vi "PIM Driver.vi"(5 "PIM Driver Name/Configuration":string, 6 "Driver Ref (null)":T1, 7 "PIM Command":T11, 8 "error in (no error)":errorcluster, 11 "Stimulus":T3={"Carrier Frequencies"={"C1 Freq, MHz"=0.0, "C2 Freq, MHz"=0.0}, "Carrier Powers"={"C1 Power,dBm"=0.0, "C2 Power, dBm"=0.0}, "Measurement Parameters"={"IM Order"=0, "Averaging"=1, "Direction"=0, "Enable ALC?"=FALSE, "Enable SingleIM?"=FALSE, "Display Units"=enum."dBm", "VA Hold?"=FALSE, "DUT PORT"=enum."Port 1"}, "Measurement Setup"={"Meas Type"=enum."Time", "TXStep"=0}} {"Measurement Setup"."TXStep" items=[".2", ".4", "1.0", "2.0"]; "Measurement Parameters"."Direction" items=["Reverse", "Forward", "Auxiliary"]; "Measurement Parameters"."IM Order" items=["3rd", "5th", "7th", "9th", "11th", "13th", "15th", "17th", "19th", "21st", "23rd", "25th", "27th", "29th", "31st", "33rd"]; "Measurement Parameters"."Averaging" items=["None", "Minimum", "Normal", "High", "Maximum"]}) -> (0 "error out":errorcluster, 2 "Variant Output":string, 3 "Measurement Results":T2 {"IMPower_dBc(s)" format="%.2f"; "TxFreqs" format="%.2f"; "IMFreq(s)" format="%.2f"; "IMPower(s)" format="%.2f"; "TxPower" format="%.2f"}, 4 "duplicate driver ref":T1)   [LabVIEW 2011]
uses:
  PIM Command.ctl
  PIM Stimulus.ctl
  PIM Cmd Params.ctl
  BPIMCore EXT/HW IO/IMOrder.ctl
  BPIMCore EXT/HW IO/HW Averaging.ctl
  BPIMCore EXT/HW IO/MeasMode.ctl
  BPIMCore EXT/Display/display_unit_format.ctl
  BPIMCore EXT/HW IO/DUTport.ctl
  BPIMCore EXT/HW IO/PIM Sweep Step Size.ctl
  PIM Results.ctl
  PIM Driver Ref.ctl
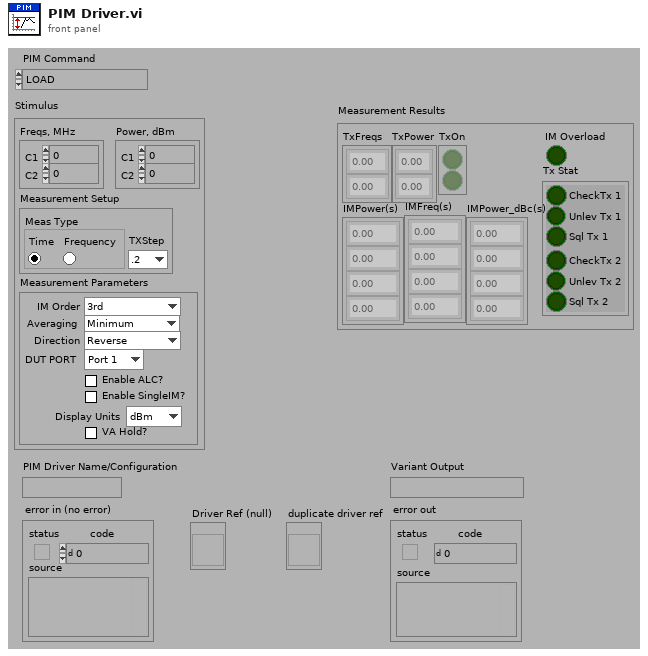
[diagram p1: front panel]
types:
  T1 = typedef "PIM Driver Ref.ctl" = refnum<vi>
  T2 = typedef "PIM Results.ctl" = cluster{"TxFreqs":dbl[], "TxPower":dbl[], "TxOn":bool[], "IMPower(s)":dbl[], "IMFreq(s)":dbl[], "Tx Stat":cluster{"CheckTx 1":bool, "Unlev Tx 1":bool, "Sql Tx 1":bool, "CheckTx 2":bool, "Unlev Tx 2":bool, "Sql Tx 2":bool}, "IM Overload":bool, "IMPower_dBc(s)":dbl[]}
  T3 = typedef "PIM Stimulus.ctl" = cluster{"Carrier Frequencies":cluster{"C1 Freq, MHz":dbl, "C2 Freq, MHz":dbl}, "Carrier Powers":cluster{"C1 Power,dBm":dbl, "C2 Power, dBm":dbl}, "Measurement Parameters":T4, "Measurement Setup":cluster{"Meas Type":enum32{"Time", "Frequency"}, "TXStep":T10}}
  T4 = typedef "PIM Cmd Params.ctl" = cluster{"IM Order":T5, "Averaging":T6, "Direction":T7, "Enable ALC?":bool, "Enable SingleIM?":bool, "Display Units":T8, "VA Hold?":bool, "DUT PORT":T9}
  T5 = typedef "IMOrder.ctl" = u8
  T6 = typedef "HW Averaging.ctl" = u16
  T7 = typedef "MeasMode.ctl" = u16
  T8 = typedef "display_unit_format.ctl" = enum16{"dBm", "dBc"}
  T9 = typedef "DUTport.ctl" = enum16{"Port 1", "Port 2"}
  T10 = typedef "PIM Sweep Step Size.ctl" = u16
  T11 = typedef "PIM Command.ctl" = enum16{"LOAD", "KEEP ALIVE", "VALIDATE", "INITIALIZE", "PRESET", "GET CALIBRATION", "SET STIMULUS", "TOGGLE TX POWER", "SET TX ON", "SET TX OFF", "MEASURE", "UNLOAD"}
  T12 = enum32{"invalid app kind", "Development System", "Run Time System", "Student Edition", "Embedded LabVIEW", "Evaluation", "Custom"}
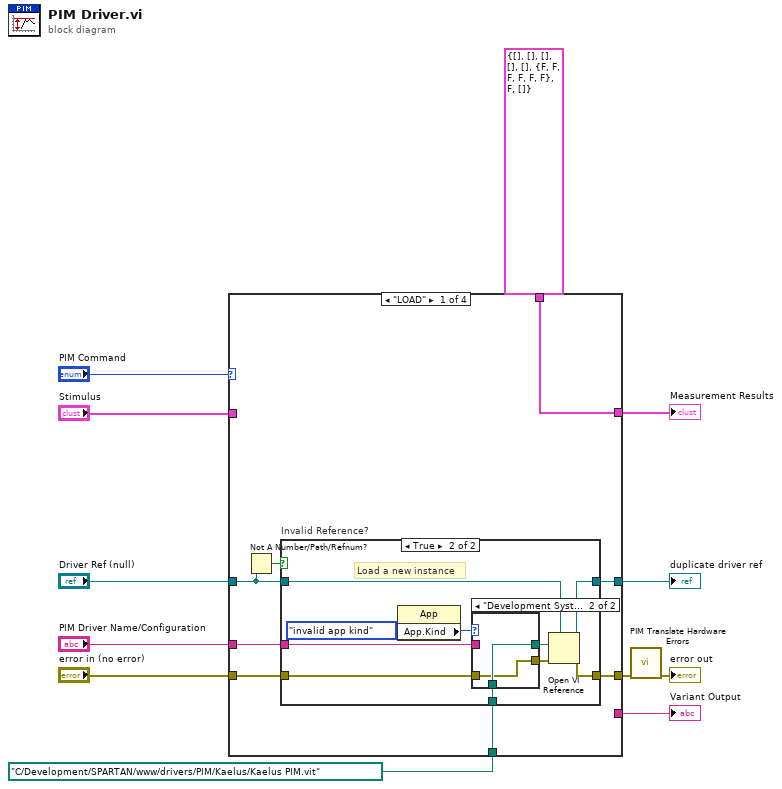
[diagram p0: block diagram]
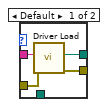
[diagram p3: hidden frame]
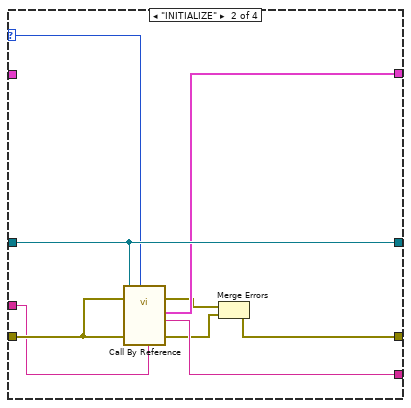
[diagram p4: hidden frame]
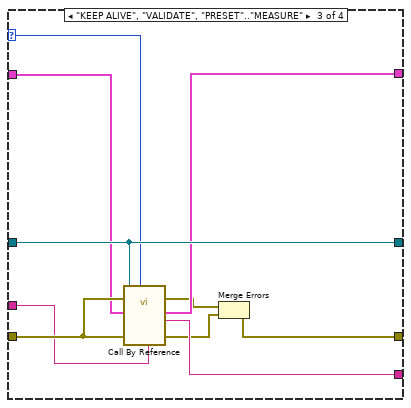
[diagram p5: hidden frame]
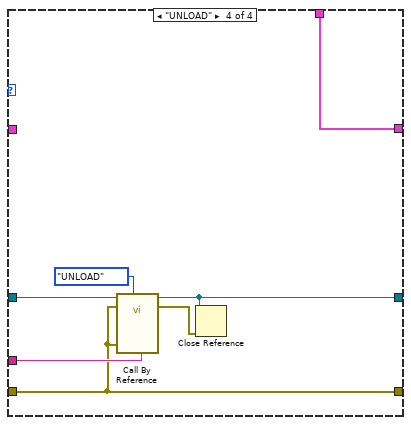
[diagram p6: hidden frame]
diagram:
  n1 = case shown="\"LOAD\"" "PIM Command" {
    selector: "PIM Command" -> [_ w41 w52 _]
    tunnel: "PIM Driver Name/Configuration" -> [w16 w42 w48 w59]
    tunnel: "error in (no error)" -> [w20 w46 w56 w57]
    tunnel: [w19 w45 w55 w57] -> w2
    tunnel: "Driver Ref (null)" -> [w15 w43 w53 w62]
    tunnel: [w17 w43 w53 w61] -> w8
    tunnel: [w18 w40 w51 w63] -> w7
    tunnel: [_ w44 w54 _] -> w6
    tunnel: "Stimulus" -> [_ _ w47 _]
    tunnel: T2 {"TxFreqs"=[], "TxPower"=[], "TxOn"=[], "IMPower(s)"=[], "IMFreq(s)"=[], "Tx Stat"={"CheckTx 1"=FALSE, "Unlev Tx 1"=FALSE, "Sql Tx 1"=FALSE, "CheckTx 2"=FALSE, "Unlev Tx 2"=FALSE, "Sql Tx 2"=FALSE}, "IM Overload"=FALSE, "IMPower_dBc(s)"=[]} ("Measurement Results") -> [w18 _ _ w63]
    tunnel: path "C:/Development/SPARTAN/www/drivers/PIM/Kaelus/Kaelus PIM.vit" ("vi path") -> [w13 _ _ _]
    frame "LOAD" {
      n2 = Not A Number/Path/Refnum?(number/path/refnum=w15) -> (NaN/Path/Refnum?=w14:bool)
      n3 = case "Invalid Reference?" shown="True" w14 {
        tunnel: w20 -> [w21 w31]
        tunnel: [w21 w30] -> w19
        tunnel: [w22 w29] -> w17
        tunnel: w16 -> [_ w28]
        tunnel: w15 -> [w22 w27]
        tunnel: w13 -> [_ w24]
        frame False {
          # "Load existing instance"
        }
        frame True {
          # "Load a new instance"
          n4 = property class="App" props=["App.Kind"]() -> ()  [unwired: 2 in, 3 out]
          n5 = case shown="\"Development System\"" T12."invalid app kind" ("App.Kind") {
            tunnel: w31 -> [w35 w36]
            tunnel: w28 -> [w34 _]
            tunnel: [w33 w36] -> w26
            tunnel: [w32 w37] -> w25
            tunnel: w24 -> [_ w37]
            frame Default {
              n6 = call "Driver Load.vi"("error in (no error)"=w35, "DriverID DriverType (\"\")"=w34) -> ("error out"=w33:errorcluster, "Driver Component Path"=w32:path)  [unwired: 1 in, 7 out]
            }
            frame "Development System" {
            }
          }
          n7 = Open VI Reference(type specifier VI Refnum (for type only)=w27, vi path=w25, error in (no error)=w26) -> (vi reference=w29:T1, error out=w30:errorcluster)  [unwired: 3 out]
        }
      }
    }
    frame "INITIALIZE" {
      n8 = call-by-ref "?"(reference=w43, error in=w46, "PIM Driver Name/Configuration"=w42, "PIM Command"=w41, "error in (no error)"=w46) -> (error out=w38:errorcluster, 0:"error out"=w39:errorcluster, "Variant Output"=w44:string, "Measurement Results"=w40:T2)  [unwired: 6 in, 1 out]
      n9 = Merge Errors(w38, w39) -> (w45:errorcluster)
    }
    frame "KEEP ALIVE", "VALIDATE", "PRESET".."MEASURE" {
      n10 = call-by-ref "?"(reference=w53, error in=w56, "PIM Driver Name/Configuration"=w48, "PIM Command"=w52, "error in (no error)"=w56, "Stimulus"=w47) -> (error out=w49:errorcluster, 0:"error out"=w50:errorcluster, "Variant Output"=w54:string, "Measurement Results"=w51:T2)  [unwired: 5 in, 1 out]
      n11 = Merge Errors(w49, w50) -> (w55:errorcluster)
    }
    frame "UNLOAD" {
      n12 = call-by-ref "?"(reference=w62, error in=w57, "PIM Driver Name/Configuration"=w59, "PIM Command"=PIM_Command."UNLOAD", "error in (no error)"=w57) -> (reference out=w61:T1, error out=w58:errorcluster)  [unwired: 6 in, 3 out]
      n13 = Close Reference(reference=w61, error in (no error)=w58) -> ()  [unwired: 1 out]
    }
  }
  "Measurement Results" <- w7
  "Variant Output" <- w6
  "duplicate driver ref" <- w8
  n14 = call "PIM Translate Hardware Errors.vi"("error in (no error)"=w2) -> ("error out"=→"error out":errorcluster)  [unwired: 10 out]
